vi "Change IP Address.vi"(0 "MAC Address in Hex":string, 2 "IP Address":string, 3 "Subnet Mask":string, 5 "Default Gateway":string) -> (6 "IP Change Frame":string)   [LabVIEW 2015]
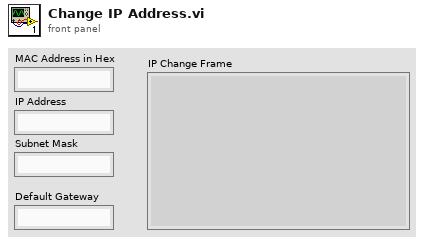
[diagram p1: front panel]
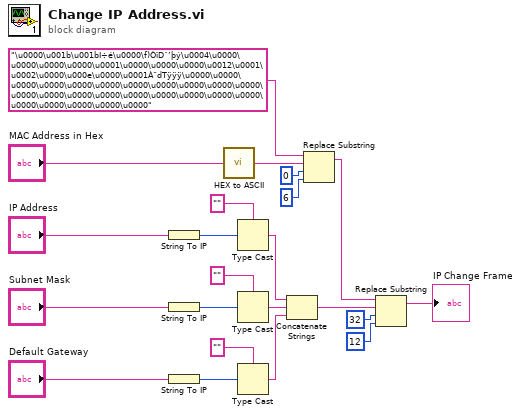
[diagram p0: block diagram]
diagram:
  n1 = String To IP(1:"IP Address") -> (0:w18:u32)
  n2 = String To IP(1:"Subnet Mask") -> (0:w16:u32)
  n3 = String To IP(1:"Default Gateway") -> (0:w14:u32)
  n4 = call "HEX to ASCII.vi"("String in HEX"="MAC Address in Hex") -> ("String in ASCII"=w21:string)
  n5 = Type Cast(type="", x=w18) -> (*(type *) &x=w12:string)
  n6 = Type Cast(type="", x=w16) -> (*(type *) &x=w10:string)
  n7 = Type Cast(type="", x=w14) -> (*(type *) &x=w11:string)
  n8 = Concatenate Strings(w12, w10, w11) -> (w8:string)
  n9 = Replace Substring(2:6 ("offset (0)"), 3:0 ("length (len. of substring)"), 4:w21, 5:"\u0000\u001b\u001bI÷é\u0000\f)ÒîDˆ’þý\u0004\u0000\u0000\u0000\u0000\u0001\u0000\u0000\u0000\u0012\u0001\u0002\u0000\u000e\u0000\u0001À¨dTÿÿÿ\u0000\u0000\u0000\u0000\u0000\u0000\u0000\u0000\u0000\u0000\u0000\u0000\u0000\u0000\u0000\u0000\u0000\u0000\u0000\u0000\u0000\u0000\u0000\u0000\u0000") -> (1:w9:string)  [unwired: 1 out]
  n10 = Replace Substring(2:12 ("length (len. of substring)"), 3:32 ("offset (0)"), 4:w8, 5:w9) -> (1:→"IP Change Frame":string)  [unwired: 1 out]
